vi "control_sas.vi"(8 "error in (no error)":errorcluster, 9 "Numeric":dbl, 10 "all rows":dbl[](array[numeric]), 11 "VISA Refnum in":refnum<visa-resource-name>) -> (0 "error out":errorcluster, 3 "VISA Refnum out":refnum<visa-resource-name>)   [LabVIEW 2019]
uses:
  <instrlib>/Agilent E4360/Agilent E4360.lvlib
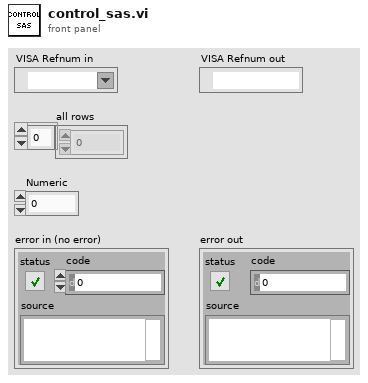
[diagram p1: front panel]
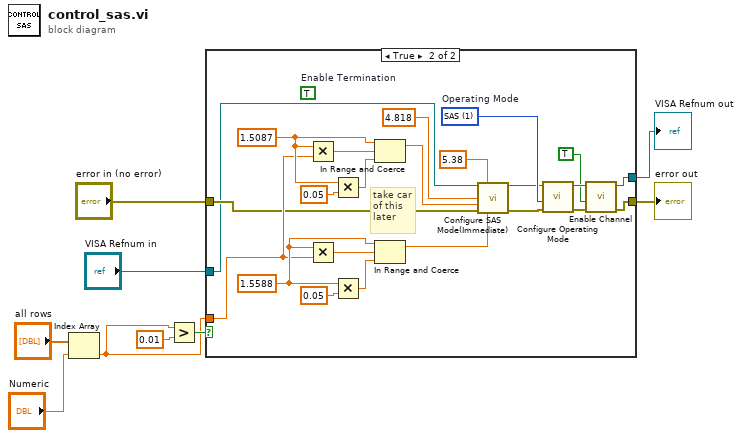
[diagram p0: block diagram]
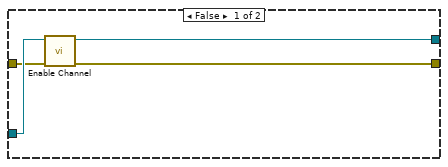
[diagram p2: hidden frame]
diagram:
  n1 = Index Array(array="all rows", index="Numeric") -> (element=w8:dbl)
  n2 = Greater?(x=w8, y=0.01) -> (0:w9:bool)
  n3 = case shown="True" w9 {
    tunnel: w8 -> [_ w18]
    tunnel: "error in (no error)" -> [w12 w17]
    tunnel: "VISA Refnum in" -> [w13 w16]
    tunnel: [w11 w15] -> w5
    tunnel: [w10 w14] -> w6
    frame False {
      n4 = call <instrlib>:"Enable Channel.vi"("error in (no error)"=w12, "VISA resource name"=w13) -> ("error out"=w10:errorcluster, "VISA resource name out"=w11:refnum<visa-resource-name>)  [unwired: 8 in]
    }
    frame True {
      w28 = 1 items=["Fixed", "SAS", "Table"]  # Operating Mode
      w19 = 1.5588 ("Maximum Current Point (0.0 A)")
      w20 = 1.5087 ("Maximum Current Point (0.0 A)")
      (unwired) TRUE  # Enable Termination
      # "take car\nof this \nlater"
      n5 = Multiply(x=w20, y=w18) -> (x*y=w22:dbl)
      n6 = Multiply(x=w19, y=w18) -> (x*y=w21:dbl)
      n7 = Multiply(x=w20, y=0.05) -> (x*y=w32:dbl)
      n8 = Multiply(x=w19, y=0.05) -> (x*y=w30:dbl)
      n9 = In Range and Coerce(upper limit=w20, x=w22, lower limit=w32) -> (coerced(x)=w34:dbl)  [unwired: 1 out]
      n10 = In Range and Coerce(upper limit=w19, x=w21, lower limit=w30) -> (coerced(x)=w29:dbl)  [unwired: 1 out]
      n11 = call <instrlib>:"Configure SAS Mode(Immediate).vi"("VISA resource name"=w16, "Open Circuit Voltage (0.0 V)"=5.38, "Maximum Voltage Point (0.0 V)"=4.818, "Maximum Current Point (0.0 A)"=w34, "error in (no error)"=w17, "Short Circuit Current (0.0 A)"=w29) -> ("VISA resource name out"=w27:refnum<visa-resource-name>, "error out"=w26:errorcluster)  [unwired: 8 in]
      n12 = call <instrlib>:"Configure Operating Mode.vi"("error in (no error)"=w26, "Operating Mode (0:Fixed)"=w28, "VISA resource name"=w27) -> ("error out"=w24:errorcluster, "VISA resource name out"=w25:refnum<visa-resource-name>)  [unwired: 7 in]
      n13 = call <instrlib>:"Enable Channel.vi"("error in (no error)"=w24, "Enable Channel (Disable)"=TRUE, "VISA resource name"=w25) -> ("error out"=w14:errorcluster, "VISA resource name out"=w15:refnum<visa-resource-name>)  [unwired: 7 in]
    }
  }
  "error out" <- w6
  "VISA Refnum out" <- w5
